vi "Test Implementatio Path.vi"(8 "error in (no error)":errorcluster, 11 "TestCase in":refnum<class "Test Osciloscope Init.lvclass">) -> (0 "error out":errorcluster, 3 "TestCase out":refnum<class "Test Osciloscope Init.lvclass">)   [LabVIEW 2020, in "Test Osciloscope Init.lvclass"]
uses:
  Test Osciloscope Init.lvclass
  <vilib>/addons/_JKI Toolkits/VI Tester/TestCase.llb/TestCase.lvclass
  C:/Program Files (x86)/National Instruments/LabVIEW 2020/vi.lib/addons/_JKI Toolkits/VI Tester/TestCase.llb/TestCase.lvclass
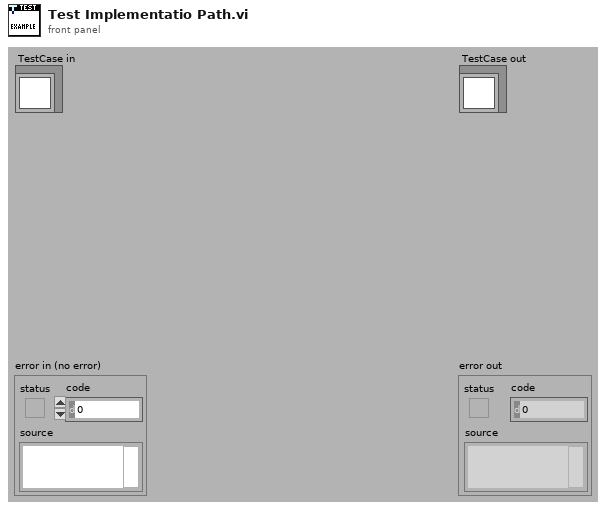
[diagram p1: front panel]
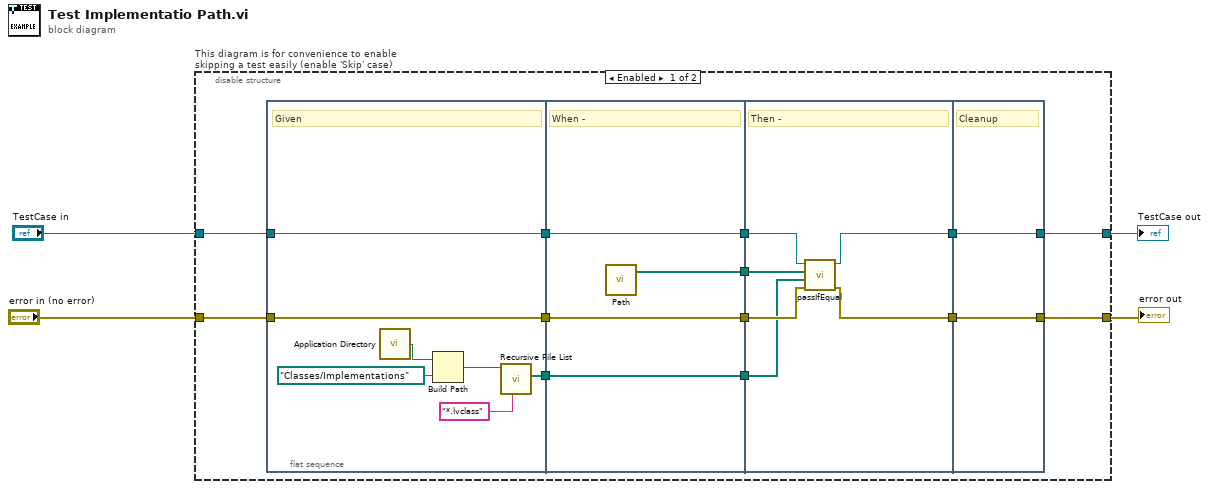
[diagram p0: block diagram]
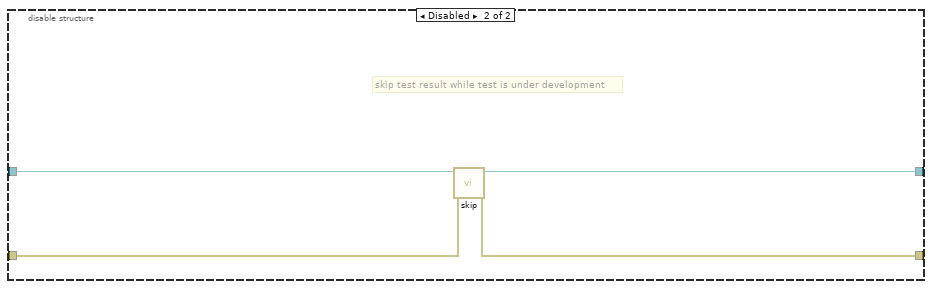
[diagram p2: hidden frame]
diagram:
  n1 = disable-structure "This diagram is for convenience to enable skipping a test easily (enable 'Skip' case)" shown="Enabled" {
    disable-tunnel: "TestCase in" -> [w11 w40]
    disable-tunnel: [w8 w38] -> w1
    disable-tunnel: [w9 w39] -> w3
    disable-tunnel: "error in (no error)" -> [w10 w37]
    frame Enabled {
      n2 = flat-sequence {
        tunnel: w10 -> [w23]
        tunnel: w11 -> [w24]
        tunnel: [w24] -> w17
        tunnel: [w23] -> w16
        tunnel: [w18] -> w5
        tunnel: [w28] -> w15
        tunnel: [w27] -> w14
        tunnel: w17 -> [w28]
        tunnel: w16 -> [w27]
        tunnel: [w26] -> w7
        tunnel: [w25] -> w6
        tunnel: w5 -> [w25]
        tunnel: [w33] -> w13
        tunnel: [w31] -> w12
        tunnel: w15 -> [w34]
        tunnel: w14 -> [w32]
        tunnel: w7 -> [w30]
        tunnel: w6 -> [w29]
        tunnel: [w35] -> w9
        tunnel: [w36] -> w8
        tunnel: w13 -> [w36]
        tunnel: w12 -> [w35]
        frame #0 {
          # "Given"
          n3 = call <vilib>:"Application Directory.vi"() -> ("Application Directory"=w19:path)
          n4 = Build Path(base path=w19, name or relative path=path "Classes/Implementations") -> (appended path=w22:path)
          n5 = call <vilib>:"Recursive File List.vi"("pattern"="*.lvclass", "Folder Path"=w22) -> ("All Files in Dir"=w18:path[])  [unwired: 5 in, 4 out]
        }
        frame #1 {
          # "When -"
          n6 = call "Path.vi"() -> ("All Files in Dir"=w26:path[])  [unwired: 11 in]
        }
        frame #2 {
          # "Then -"
          n7 = call-dynamic "passIfEqual.vi"("error in (no error)"=w32, "y"=w29, "x"=w30, "TestCase in"=w34) -> ("error out"=w31:errorcluster, "TestCase out"=w33:refnum<class "Test Osciloscope Init.lvclass">)  [unwired: 6 in]
        }
        frame #3 {
          # "Cleanup"
        }
      }
    }
    frame Disabled {
      # "skip test result while test is under development"
      n8 = call <vilib>:"skip.vi"("error in (no error)"=w37, "TestCase in"=w40) -> ("error out"=w39:errorcluster, "TestCase out"=w38:refnum<class "Test Osciloscope Init.lvclass">)  [unwired: 8 in]
    }
  }
  "error out" <- w3
  "TestCase out" <- w1
